vi "Manual_batch_DCIMG_to_TIFF_conversion_single_color_only.vi"() -> ()   [LabVIEW 2016]
panel:
  out "Numeric":i32
  in  "Select dataset folder":path
  out "size(s)":i32
  out "error IO":errorcluster
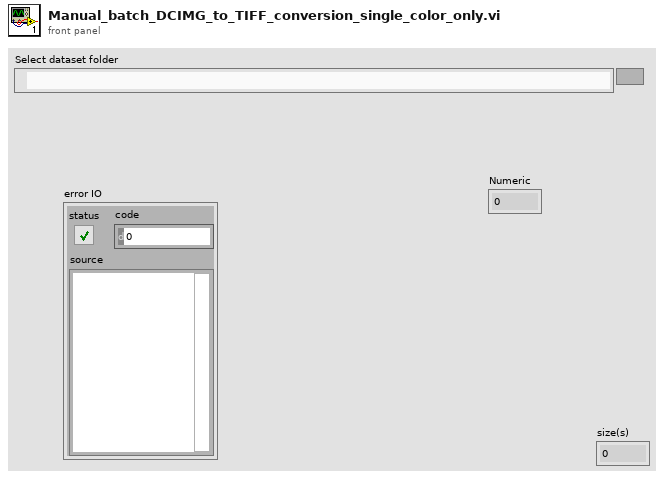
[diagram p1: front panel]
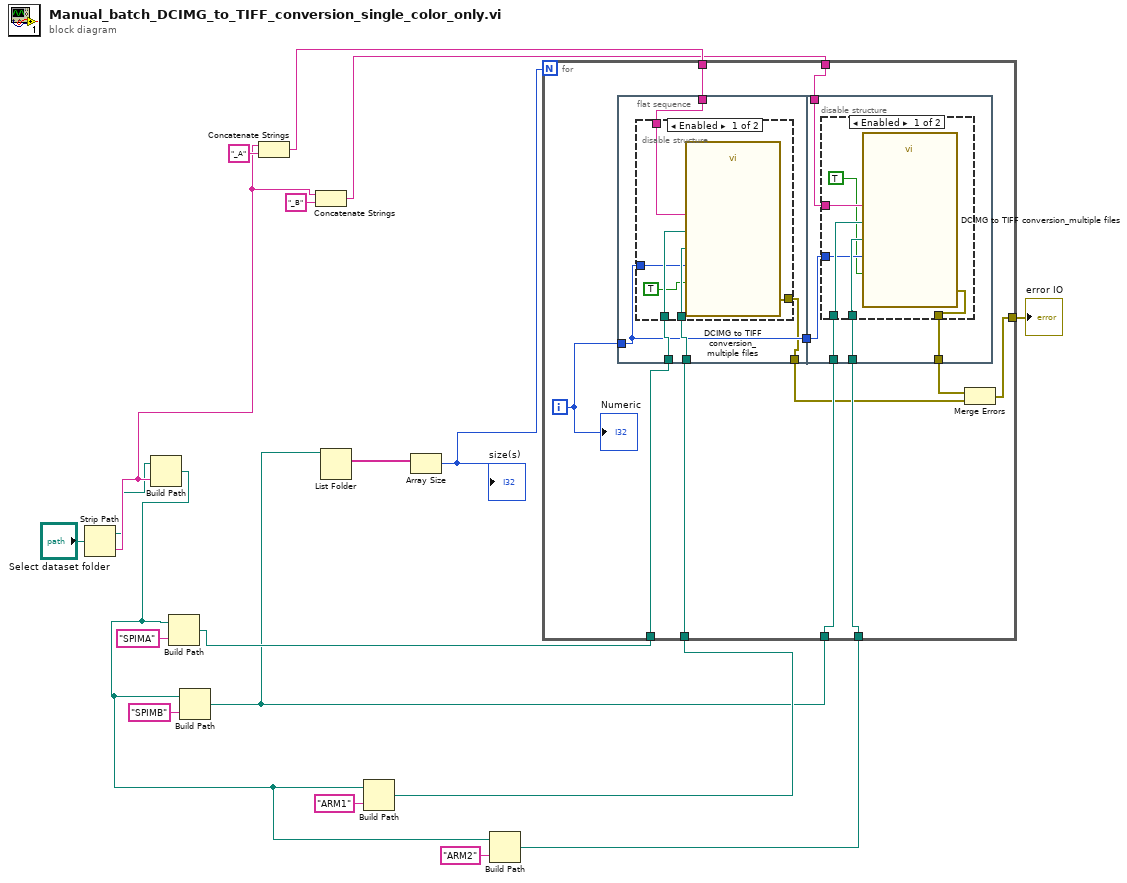
[diagram p0: block diagram]
diagram:
  n1 = Strip Path(path="Select dataset folder") -> (stripped path=w2:path, name=w3:string)
  n2 = Build Path(base path=w2, name or relative path=w3) -> (appended path=w9:path)
  n3 = Build Path(base path=w9, name or relative path="SPIMA") -> (appended path=w6:path)
  n4 = Build Path(base path=w9, name or relative path="SPIMB") -> (appended path=w1:path)
  n5 = Concatenate Strings(w3, "_A" ("string")) -> (w14:string)
  n6 = Concatenate Strings(w3, "_B" ("string")) -> (w12:string)
  n7 = List Folder(path=w1) -> (filenames=w19:string[])  [unwired: 3 in, 3 out]
  n8 = Build Path(base path=w9, name or relative path="ARM1") -> (appended path=w10:path)
  n9 = Array Size(array=w19) -> (size(s)=w5:i32)
  "size(s)" <- w5
  n10 = Build Path(base path=w9, name or relative path="ARM2") -> (appended path=w7:path)
  n11 = for {
    N: w5 -> [_]
    tunnel: w6 -> [w30]
    tunnel: w1 -> [w29]
    tunnel: [w22] -> w18
    tunnel: w10 -> [w28]
    tunnel: w7 -> [w27]
    tunnel: w14 -> [w21]
    tunnel: w12 -> [w20]
    i -> [w26]
    n12 = flat-sequence {
      tunnel: w30 -> [w35]
      tunnel: w26 -> [w33]
      tunnel: w28 -> [w34]
      tunnel: [w33] -> w25
      tunnel: [w32] -> w23
      tunnel: w21 -> [w31]
      tunnel: w29 -> [w46]
      tunnel: w27 -> [w45]
      tunnel: w25 -> [w44]
      tunnel: [w43] -> w24
      tunnel: w20 -> [w42]
      frame #0 {
        n13 = disable-structure shown="Enabled" {
          disable-tunnel: w35 -> [w41 _]
          disable-tunnel: w34 -> [w40 _]
          disable-tunnel: w33 -> [w39 _]
          disable-tunnel: [w38 _] -> w32
          disable-tunnel: w31 -> [w37 _]
          frame Enabled {
            n14 = call "DCIMG to TIFF conversion_multiple files.vi"("Volume number"=w39, "IsSingleColor"=TRUE, "Input File Path"=w41, "Input File Name"=w37, "Output Path"=w40) -> ("Error Out"=w38:errorcluster)  [unwired: 5 in, 5 out]
          }
          frame Disabled {
          }
        }
      }
      frame #1 {
        n15 = disable-structure shown="Enabled" {
          disable-tunnel: w46 -> [w52 _]
          disable-tunnel: w45 -> [w51 _]
          disable-tunnel: w44 -> [w50 _]
          disable-tunnel: [w49 _] -> w43
          disable-tunnel: w42 -> [w48 _]
          frame Enabled {
            n16 = call "DCIMG to TIFF conversion_multiple files.vi"("Volume number"=w50, "IsSingleColor"=TRUE, "Input File Path"=w52, "Input File Name"=w48, "Output Path"=w51) -> ("Error Out"=w49:errorcluster)  [unwired: 5 in, 5 out]
          }
          frame Disabled {
          }
        }
      }
    }
    n17 = Merge Errors(w24, w23) -> (w22:errorcluster)
    "Numeric" <- w26
  }
  "error IO" <- w18
